vi "LDA+_An_Analysis_mode.vi"(6 "Second Graph":T2={"Plot 1"=1, "Plot 2"=2, "Save graph"=0, "Plot Type"=enum."Voltage trace"} {"Save graph" items=["Do not save plot", "Save plot"]; "Plot 2" items=["Nothing", "Prop 2 (U)"]; "Plot 1" items=["Nothing", "Prop 2 (U)"]}, 9 "First Graph":T2={"Plot 1"=1, "Plot 2"=2, "Save graph"=0, "Plot Type"=enum."Voltage trace"} {"Save graph" items=["Do not save plot", "Save plot"]; "Plot 2" items=["Nothing", "Prop 2 (U)"]; "Plot 1" items=["Nothing", "Prop 2 (U)"]}) -> (0 "Second Graph out":T2={"Plot 1"=1, "Plot 2"=2, "Save graph"=0, "Plot Type"=enum."Voltage trace"} {"Save graph" items=["Do not save plot", "Save plot"]; "Plot 2" items=["Nothing", "Prop 2 (U)"]; "Plot 1" items=["Nothing", "Prop 2 (U)"]}, 3 "First Graph out":T2={"Plot 1"=1, "Plot 2"=2, "Save graph"=0, "Plot Type"=enum."Voltage trace"} {"Save graph" items=["Do not save plot", "Save plot"]; "Plot 2" items=["Nothing", "Prop 2 (U)"]; "Plot 1" items=["Nothing", "Prop 2 (U)"]})   [LabVIEW 2010]
uses:
  Controls/Graph_Type.ctl
  Globals/Meas_global.vi
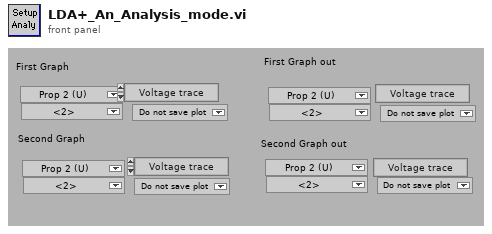
[diagram p1: front panel]
types:
  T1 = typedef "Graph_Type.ctl" = enum16{"Show no graph", "Voltage trace", "Velocity trace", "Vel histogram", "Spectrum", "f.E(f) v Log f", "Auto-Corr"}
  T2 = cluster{"Plot 1":u16, "Plot 2":u16, "Save graph":u16, "Plot Type":T1}
  T3 = typedef "Analysis_info_cluster.ctl" = cluster{"Colour":u32, "Inst type":T4, "Inst name":string, "Symbol":string, "Code name":string, "Extra Info":string, "Inst Array":T5, "Index":i32, "Voltage Index":i32, "Extra Titles":string[], "Extra Values":string[]}
  T4 = typedef "Inst_type.ctl" = enum16{"Propeller anemometer", "Raw voltage", "Pressure Transducer", "Pitot-static tube", "Preston tube", "Hot wire", "Cross wire 1", "Cross wire 2", "Generic Linear", "Generic Polynomial", "Generic BackPoly", "Fast FID", "Thermocouple", "Cold wire", "Pulsed Wire", "LDA Vel", "LDA Tran time", "LDA Arr time"}
  T5 = typedef "Instrument_Array.ctl" = enum16{"PWA", "LDA", "Analogue"}
  T6 = enum16{"Show no graph", "Voltage trace", "Velocity trace", " Vel histogram", "Spectrum", "f.E(f) v Log f", "Auto-Corr"}
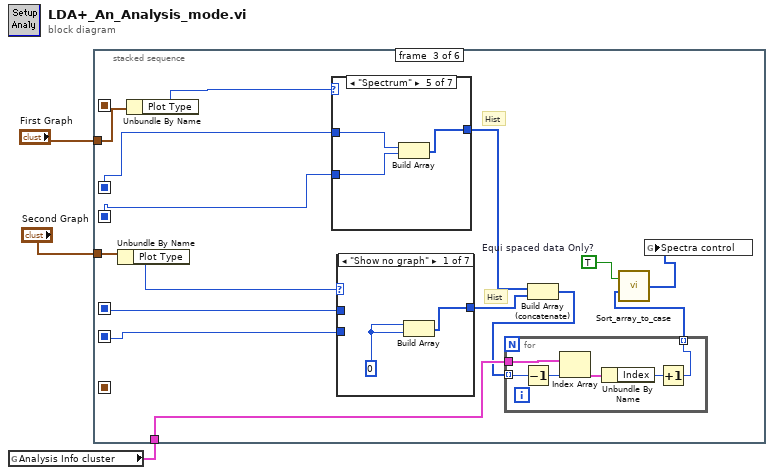
[diagram p0: block diagram]
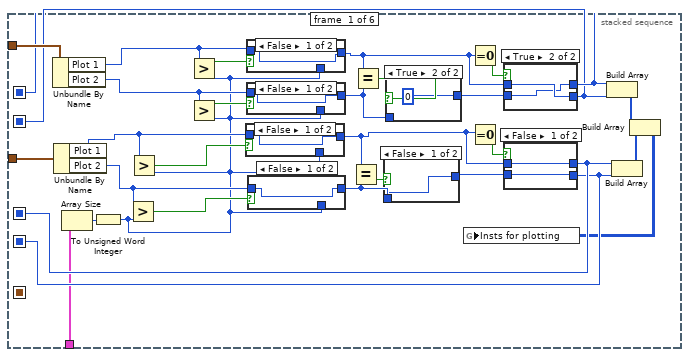
[diagram p2: hidden frame]
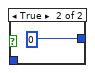
[diagram p10: hidden frame]
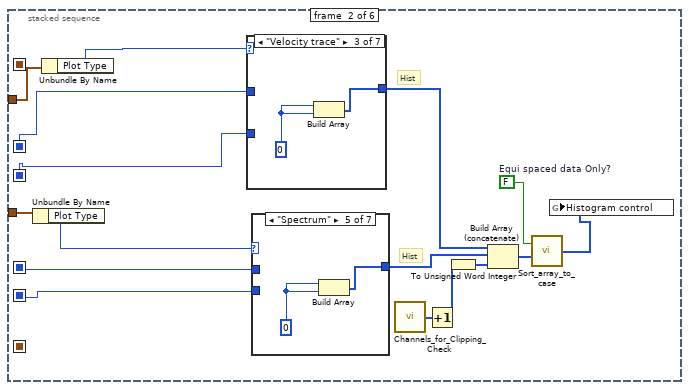
[diagram p11: hidden frame]
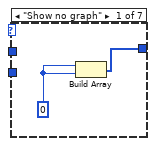
[diagram p12: hidden frame]
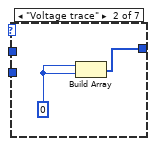
[diagram p13: hidden frame]
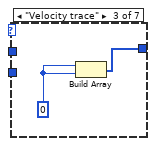
[diagram p14: hidden frame]
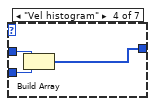
[diagram p15: hidden frame]
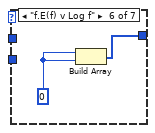
[diagram p16: hidden frame]
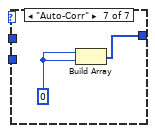
[diagram p17: hidden frame]
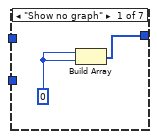
[diagram p18: hidden frame]
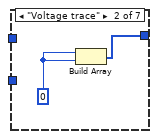
[diagram p19: hidden frame]
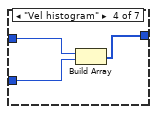
[diagram p20: hidden frame]
diagram:
  n1 = global read "Meas_global.vi" "Analysis Info cluster"() -> (w1:T3[])
  n2 = stacked-sequence {
    seq-local: [w15 _ _ _ _ _] -> [_ w64 w110 w163 w209 _]
    seq-local: [w14 _ _ _ _ _] -> [_ w63 w109 w162 w208 _]
    seq-local: [w10 _ _ _ _ _] -> [_ w66 w112 w165 w203 _]
    seq-local: [w9 _ _ _ _ _] -> [_ w65 w111 w164 w202 _]
    seq-local: [_ _ _ _ w199 _] -> [_ _ _ _ _ w237]
    seq-local: [_ _ _ _ w200 _] -> [_ _ _ _ _ w233]
    tunnel: "First Graph" -> [w24 w62 w108 w161 w212 _]
    tunnel: "Second Graph" -> [w23 w61 w107 w160 w206 _]
    tunnel: w1 -> [w4 _ w102 _ _ _]
    frame #0 {
      n3 = Unbundle By Name(w24) -> ("Plot 1"=w22:u16, "Plot 2"=w21:u16)
      n4 = Unbundle By Name(w23) -> ("Plot 1"=w20:u16, "Plot 2"=w19:u16)
      n5 = Array Size(array=w4) -> (size(s)=w33:i32)
      n6 = To Unsigned Word Integer(number=w33) -> (unsigned 16bit integer=w5:u16)
      n7 = Greater?(x=w19, y=w5) -> (0:w29:bool)
      n8 = Greater?(x=w20, y=w5) -> (0:w28:bool)
      n9 = Greater?(x=w22, y=w5) -> (0:w26:bool)
      n10 = Greater?(x=w21, y=w5) -> (0:w27:bool)
      n11 = case shown="False" w28 {
        tunnel: [w48 w49] -> w12
        tunnel: w20 -> [w48 _]
        tunnel: w5 -> [_ w49]
        frame False {
        }
        frame True {
        }
      }
      n12 = case shown="False" w26 {
        tunnel: [w44 w45] -> w17
        tunnel: w22 -> [w44 _]
        tunnel: w5 -> [_ w45]
        frame False {
        }
        frame True {
        }
      }
      n13 = case shown="False" w27 {
        tunnel: [w46 w47] -> w30
        tunnel: w21 -> [w46 _]
        tunnel: w5 -> [_ w47]
        frame False {
        }
        frame True {
        }
      }
      n14 = case shown="False" w29 {
        tunnel: [w50 w51] -> w32
        tunnel: w19 -> [w50 _]
        tunnel: w5 -> [_ w51]
        frame False {
        }
        frame True {
        }
      }
      n15 = Equal?(x=w12, y=w32) -> (x = y?=w31:bool)
      n16 = Equal?(x=w17, y=w30) -> (x = y?=w25:bool)
      n17 = case shown="False" w31 {
        tunnel: [w52 u16 0] -> w11
        tunnel: w32 -> [w52 _]
        frame False {
        }
        frame True {
        }
      }
      n18 = case shown="True" w25 {
        tunnel: [w42 u16 0] -> w16
        tunnel: w30 -> [w42 _]
        frame False {
        }
        frame True {
        }
      }
      n19 = Equal To 0?(x=w17) -> (x = 0?=w18:bool)
      n20 = Equal To 0?(x=w12) -> (x = 0?=w13:bool)
      n21 = case shown="True" w18 {
        tunnel: [w38 w41] -> w14
        tunnel: w17 -> [w39 w41]
        tunnel: [w39 w40] -> w15
        tunnel: w16 -> [w38 w40]
        frame False {
        }
        frame True {
        }
      }
      n22 = case shown="False" w13 {
        tunnel: [w34 w37] -> w9
        tunnel: w12 -> [w35 w37]
        tunnel: [w35 w36] -> w10
        tunnel: w11 -> [w34 w36]
        frame False {
        }
        frame True {
        }
      }
      n23 = Build Array(w15, w14) -> (w8:u16[])
      n24 = Build Array(w10, w9) -> (w7:u16[])
      n25 = Build Array(w8, w7) -> (w6:u16[][])
      n26 = global write "Meas_global.vi" "Insts for plotting"(w6) -> ()
    }
    frame #1 {
      w54 = FALSE  # Equi spaced data Only?
      # "Hist"
      # "Hist"
      n27 = Unbundle By Name(w61) -> ("Plot Type"=w59:T1)
      n28 = Unbundle By Name(w62) -> ("Plot Type"=w60:T1)
      n29 = case shown="\"Velocity trace\"" w60 {
        tunnel: w64 -> [_ _ _ w92 _ _ _]
        tunnel: w63 -> [_ _ _ w91 _ _ _]
        tunnel: [w85 w87 w89 w93 w94 w96 w98] -> w69
        frame "Show no graph" {
          w86 = u16 0
          n30 = Build Array(w86, w86) -> (w85:u16[])
        }
        frame "Voltage trace" {
          w88 = u16 0
          n31 = Build Array(w88, w88) -> (w87:u16[])
        }
        frame "Velocity trace" {
          w90 = u16 0
          n32 = Build Array(w90, w90) -> (w89:u16[])
        }
        frame "Vel histogram" {
          n33 = Build Array(w92, w91) -> (w93:u16[])
        }
        frame "Spectrum" {
          w95 = u16 0
          n34 = Build Array(w95, w95) -> (w94:u16[])
        }
        frame "f.E(f) v Log f" {
          w97 = u16 0
          n35 = Build Array(w97, w97) -> (w96:u16[])
        }
        frame "Auto-Corr" {
          w99 = u16 0
          n36 = Build Array(w99, w99) -> (w98:u16[])
        }
      }
      n37 = case shown="\"Spectrum\"" w59 {
        tunnel: w66 -> [_ _ _ w78 _ _ _]
        tunnel: w65 -> [_ _ _ w77 _ _ _]
        tunnel: [w70 w72 w74 w76 w79 w81 w83] -> w68
        frame "Show no graph" {
          w71 = u16 0
          n38 = Build Array(w71, w71) -> (w70:u16[])
        }
        frame "Voltage trace" {
          w73 = u16 0
          n39 = Build Array(w73, w73) -> (w72:u16[])
        }
        frame "Velocity trace" {
          w75 = u16 0
          n40 = Build Array(w75, w75) -> (w74:u16[])
        }
        frame "Vel histogram" {
          n41 = Build Array(w78, w77) -> (w76:u16[])
        }
        frame "Spectrum" {
          w80 = u16 0
          n42 = Build Array(w80, w80) -> (w79:u16[])
        }
        frame "f.E(f) v Log f" {
          w82 = u16 0
          n43 = Build Array(w82, w82) -> (w81:u16[])
        }
        frame "Auto-Corr" {
          w84 = u16 0
          n44 = Build Array(w84, w84) -> (w83:u16[])
        }
      }
      n45 = call "Channels_for_Clipping_Check.vi"() -> ("Channel Indicies"=w57:i32[])
      n46 = Increment(x=w57) -> (x+1=w55:i32[])
      n47 = To Unsigned Word Integer(number=w55) -> (unsigned 16bit integer=w56:u16[])
      n48 = Build Array (concatenate)(w69, w68, w56) -> (w67:u16[])
      n49 = call "Sort_array_to_case.vi"("Array to sort"=w67, "Equi spaced data Only?"=w54) -> ("Sorted Array"=w58:i32[])
      n50 = global write "Meas_global.vi" "Histogram control"(w58) -> ()
    }
    frame #2 {
      w103 = TRUE  # Equi spaced data Only?
      # "Hist"
      # "Hist"
      n51 = Unbundle By Name(w107) -> ("Plot Type"=w105:T1)
      n52 = Unbundle By Name(w108) -> ("Plot Type"=w106:T1)
      n53 = case shown="\"Spectrum\"" w106 {
        tunnel: w110 -> [_ _ _ _ w146 w149 _]
        tunnel: w109 -> [_ _ _ _ w145 w148 _]
        tunnel: [w137 w139 w141 w143 w147 w150 w151] -> w114
        frame "Show no graph" {
          w138 = u16 0
          n54 = Build Array(w138, w138) -> (w137:u16[])
        }
        frame "Voltage trace" {
          w140 = u16 0
          n55 = Build Array(w140, w140) -> (w139:u16[])
        }
        frame "Velocity trace" {
          w142 = u16 0
          n56 = Build Array(w142, w142) -> (w141:u16[])
        }
        frame "Vel histogram" {
          w144 = u16 0
          n57 = Build Array(w144, w144) -> (w143:u16[])
        }
        frame "Spectrum" {
          n58 = Build Array(w146, w145) -> (w147:u16[])
        }
        frame "f.E(f) v Log f" {
          n59 = Build Array(w149, w148) -> (w150:u16[])
        }
        frame "Auto-Corr" {
          w152 = u16 0
          n60 = Build Array(w152, w152) -> (w151:u16[])
        }
      }
      n61 = case shown="\"Show no graph\"" w105 {
        tunnel: w112 -> [_ _ _ _ w131 w134 _]
        tunnel: w111 -> [_ _ _ _ w130 w133 _]
        tunnel: [w121 w123 w125 w127 w129 w132 w135] -> w113
        frame "Show no graph" {
          w122 = u16 0
          n62 = Build Array(w122, w122) -> (w121:u16[])
        }
        frame "Voltage trace" {
          w124 = u16 0
          n63 = Build Array(w124, w124) -> (w123:u16[])
        }
        frame "Velocity trace" {
          w126 = u16 0
          n64 = Build Array(w126, w126) -> (w125:u16[])
        }
        frame "Vel histogram" {
          w128 = u16 0
          n65 = Build Array(w128, w128) -> (w127:u16[])
        }
        frame "Spectrum" {
          n66 = Build Array(w131, w130) -> (w129:u16[])
        }
        frame "f.E(f) v Log f" {
          n67 = Build Array(w134, w133) -> (w132:u16[])
        }
        frame "Auto-Corr" {
          w136 = u16 0
          n68 = Build Array(w136, w136) -> (w135:u16[])
        }
      }
      n69 = Build Array (concatenate)(w114, w113) -> (w101:u16[])
      n70 = for {
        tunnel: w101 -> [w117] mode=indexing
        tunnel: w102 -> [w120]
        tunnel: [w115] -> w100 mode=indexing
        n71 = Decrement(x=w117) -> (x-1=w118:u16)
        n72 = Index Array(array=w120, index=w118) -> (element=w119:T3)
        n73 = Unbundle By Name(w119) -> ("Index"=w116:i32)
        n74 = Increment(x=w116) -> (x+1=w115:i32)
      }
      n75 = call "Sort_array_to_case.vi"("Array to sort"=w100, "Equi spaced data Only?"=w103) -> ("Sorted Array"=w104:i32[])
      n76 = global write "Meas_global.vi" "Spectra control"(w104) -> ()
    }
    frame #3 {
      w156 = TRUE  # Equi spaced data Only?
      # "Hist"
      # "Hist"
      n77 = Unbundle By Name(w160) -> ("Plot Type"=w158:T1)
      n78 = Unbundle By Name(w161) -> ("Plot Type"=w159:T1)
      n79 = case shown="\"Auto-Corr\"" w159 {
        tunnel: w163 -> [_ _ _ _ _ _ w197]
        tunnel: w162 -> [_ _ _ _ _ _ w196]
        tunnel: [w184 w186 w188 w190 w192 w194 w198] -> w168
        frame "Show no graph" {
          w185 = u16 0
          n80 = Build Array(w185, w185) -> (w184:u16[])
        }
        frame "Voltage trace" {
          w187 = u16 0
          n81 = Build Array(w187, w187) -> (w186:u16[])
        }
        frame "Velocity trace" {
          w189 = u16 0
          n82 = Build Array(w189, w189) -> (w188:u16[])
        }
        frame "Vel histogram" {
          w191 = u16 0
          n83 = Build Array(w191, w191) -> (w190:u16[])
        }
        frame "Spectrum" {
          w193 = u16 0
          n84 = Build Array(w193, w193) -> (w192:u16[])
        }
        frame "f.E(f) v Log f" {
          w195 = u16 0
          n85 = Build Array(w195, w195) -> (w194:u16[])
        }
        frame "Auto-Corr" {
          n86 = Build Array(w197, w196) -> (w198:u16[])
        }
      }
      n87 = case shown="\"Show no graph\"" w158 {
        tunnel: w165 -> [_ _ _ _ _ _ w183]
        tunnel: w164 -> [_ _ _ _ _ _ w182]
        tunnel: [w169 w171 w173 w175 w177 w179 w181] -> w167
        frame "Show no graph" {
          w170 = u16 0
          n88 = Build Array(w170, w170) -> (w169:u16[])
        }
        frame "Voltage trace" {
          w172 = u16 0
          n89 = Build Array(w172, w172) -> (w171:u16[])
        }
        frame "Velocity trace" {
          w174 = u16 0
          n90 = Build Array(w174, w174) -> (w173:u16[])
        }
        frame "Vel histogram" {
          w176 = u16 0
          n91 = Build Array(w176, w176) -> (w175:u16[])
        }
        frame "Spectrum" {
          w178 = u16 0
          n92 = Build Array(w178, w178) -> (w177:u16[])
        }
        frame "f.E(f) v Log f" {
          w180 = u16 0
          n93 = Build Array(w180, w180) -> (w179:u16[])
        }
        frame "Auto-Corr" {
          n94 = Build Array(w183, w182) -> (w181:u16[])
        }
      }
      n95 = call "Timescale_Check.vi"() -> ("Channel Indicies"=w154:i32[])
      n96 = Increment(x=w154) -> (x+1=w155:i32[])
      n97 = To Unsigned Word Integer(number=w155) -> (unsigned 16bit integer=w153:u16[])
      n98 = Build Array (concatenate)(w168, w167, w153) -> (w166:u16[])
      n99 = call "Sort_array_to_case.vi"("Array to sort"=w166, "Equi spaced data Only?"=w156) -> ("Sorted Array"=w157:i32[])
      n100 = global write "Meas_global.vi" "Auto-Corr control"(w157) -> ()
    }
    frame #4 {
      n101 = Equal To 0?(x=w202) -> (x = 0?=w205:bool)
      n102 = Equal To 0?(x=w203) -> (x = 0?=w204:bool)
      n103 = Equal To 0?(x=w208) -> (x = 0?=w210:bool)
      n104 = Equal To 0?(x=w209) -> (x = 0?=w211:bool)
      n105 = And(x=w204, y=w205) -> (x .and. y?=w201:bool)
      n106 = And(x=w211, y=w210) -> (x .and. y?=w207:bool)
      n107 = case shown="False" w201 {
        tunnel: [w216 w221] -> w200
        tunnel: w202 -> [w215 w220]
        tunnel: w203 -> [w214 w219]
        tunnel: w206 -> [w213 w218]
        frame False {
          n108 = Bundle By Name(cluster=w213, "Plot 1"=w214, "Plot 2"=w215) -> (w216:T2)
        }
        frame True {
          n109 = Bundle By Name(cluster=w218, "Plot 1"=w219, "Plot 2"=w220, "Save graph"=0) -> (w221:T2)
        }
      }
      n110 = case shown="True" w207 {
        tunnel: [w225 w230] -> w199
        tunnel: w208 -> [w224 w229]
        tunnel: w209 -> [w223 w228]
        tunnel: w212 -> [w222 w227]
        frame False {
          n111 = Bundle By Name(cluster=w222, "Plot 1"=w223, "Plot 2"=w224) -> (w225:T2)
        }
        frame True {
          n112 = Bundle By Name(cluster=w227, "Plot 1"=w228, "Plot 2"=w229, "Save graph"=0) -> (w230:T2)
        }
      }
    }
    frame #5 {
      w232 = T6."Show no graph" ("Plot Type")
      n113 = Unbundle By Name(w233) -> ("Plot Type"=w234:T1)
      n114 = Unbundle By Name(w237) -> ("Plot Type"=w239:T1)
      n115 = Equal?(x=w239, y=w232) -> (x = y?=w238:bool)
      n116 = Equal?(x=w234, y=w232) -> (x = y?=w235:bool)
      n117 = case shown="True" w238 {
        tunnel: w237 -> [w244 w247]
        tunnel: [w244 w245] -> w236
        frame False {
        }
        frame True {
          n118 = Bundle By Name(cluster=w247, "Save graph"=u16 0) -> (w245:T2)
        }
      }
      "First Graph out" <- w236
      n119 = case shown="True" w235 {
        tunnel: w233 -> [w240 w243]
        tunnel: [w240 w241] -> w231
        frame False {
        }
        frame True {
          n120 = Bundle By Name(cluster=w243, "Save graph"=u16 0) -> (w241:T2)
        }
      }
      "Second Graph out" <- w231
    }
  }
